vi "cRIO_v5.vi"() -> ()   [LabVIEW 2015]
uses:
  <vilib>/FPGAPlugInAG/cRIO-9113/niLvFpga_Open_cRIO-9113.vi
  <vilib>/rvi/interface/common/dynamic/niFpgaDynamicAddResources.vi
  <vilib>/Utility/error.llb/Error Cluster From Error Code.vi
  <vilib>/FPGAPlugInAG/Dynamic/niLvFpga_Run_Dynamic.vi
  <vilib>/rvi/interface/common/niFpgaWaitOnOcc.vi
  <vilib>/rvi/errors/niLvFpgaAdjustHostInterfaceError.vi
  <vilib>/FPGAPlugInAG/Dynamic/niLvFpga_Close_Dynamic.vi
  <vilib>/rvi/interface/nirviOpenFPGA/nirviOpenFPGA.xnode
  FPGA Bitfiles/DW40ticks_FPGATarget_Fpgav8_YeJ2LnDYWYw.lvbitx
  Fpga_v8.vi
  <vilib>/rvi/interface/nirviMethod/nirviMethod.xnode
  <vilib>/rvi/interface/nirviReadWriteControl/nirviReadWriteControl.xnode
  <vilib>/rvi/interface/nirviCloseFPGA/nirviCloseFPGA.xnode
  <vilib>/rvi/errors/niLvFpgaMergeErrorWithErrorCode.vi
  <vilib>/FPGAPlugInAG/Dynamic/niLvFpga_ReadFifo_Dynamic.vi
  <vilib>/rvi/interface/Simulation/niFpgaSimulationCallBeginRW.vi
  NiFpgaLv.dll
  <vilib>/FPGAPlugInAG/Dynamic/niLvFpga_StartFifo_Dynamic.vi
  <vilib>/FPGAPlugInAG/Dynamic/niLvFpga_ConfigureFifo_Dynamic.vi
panel:
  out "Waveform Graph 4":sgl[](graph)
  out "Waveform Graph 3":sgl[](graph)
  out "Waveform Graph 2":sgl[](graph)
  out "decimated array":i32[](array[numeric])
  out "Analog Input Chart":sgl[][](graph)
  out "Gauge":i16
  out "Aquisition loop rate":u32
  out "error out":errorcluster
  out "Actual Depth of FIFO":u32
  out "Initial write Elements Remaining":u32
  in  "stop":bool
  out "Timed Out?":bool
  out "Number of times timed out":u8
  out "backlog (Elements remaing on the write)":u32
  out "Waveform Graph":sgl[][](graph)
  in  "Data write ON/OFF":bool
  out "Time(ms) for a loop":u32
  in  "start":bool
  out "x-y 3":u32
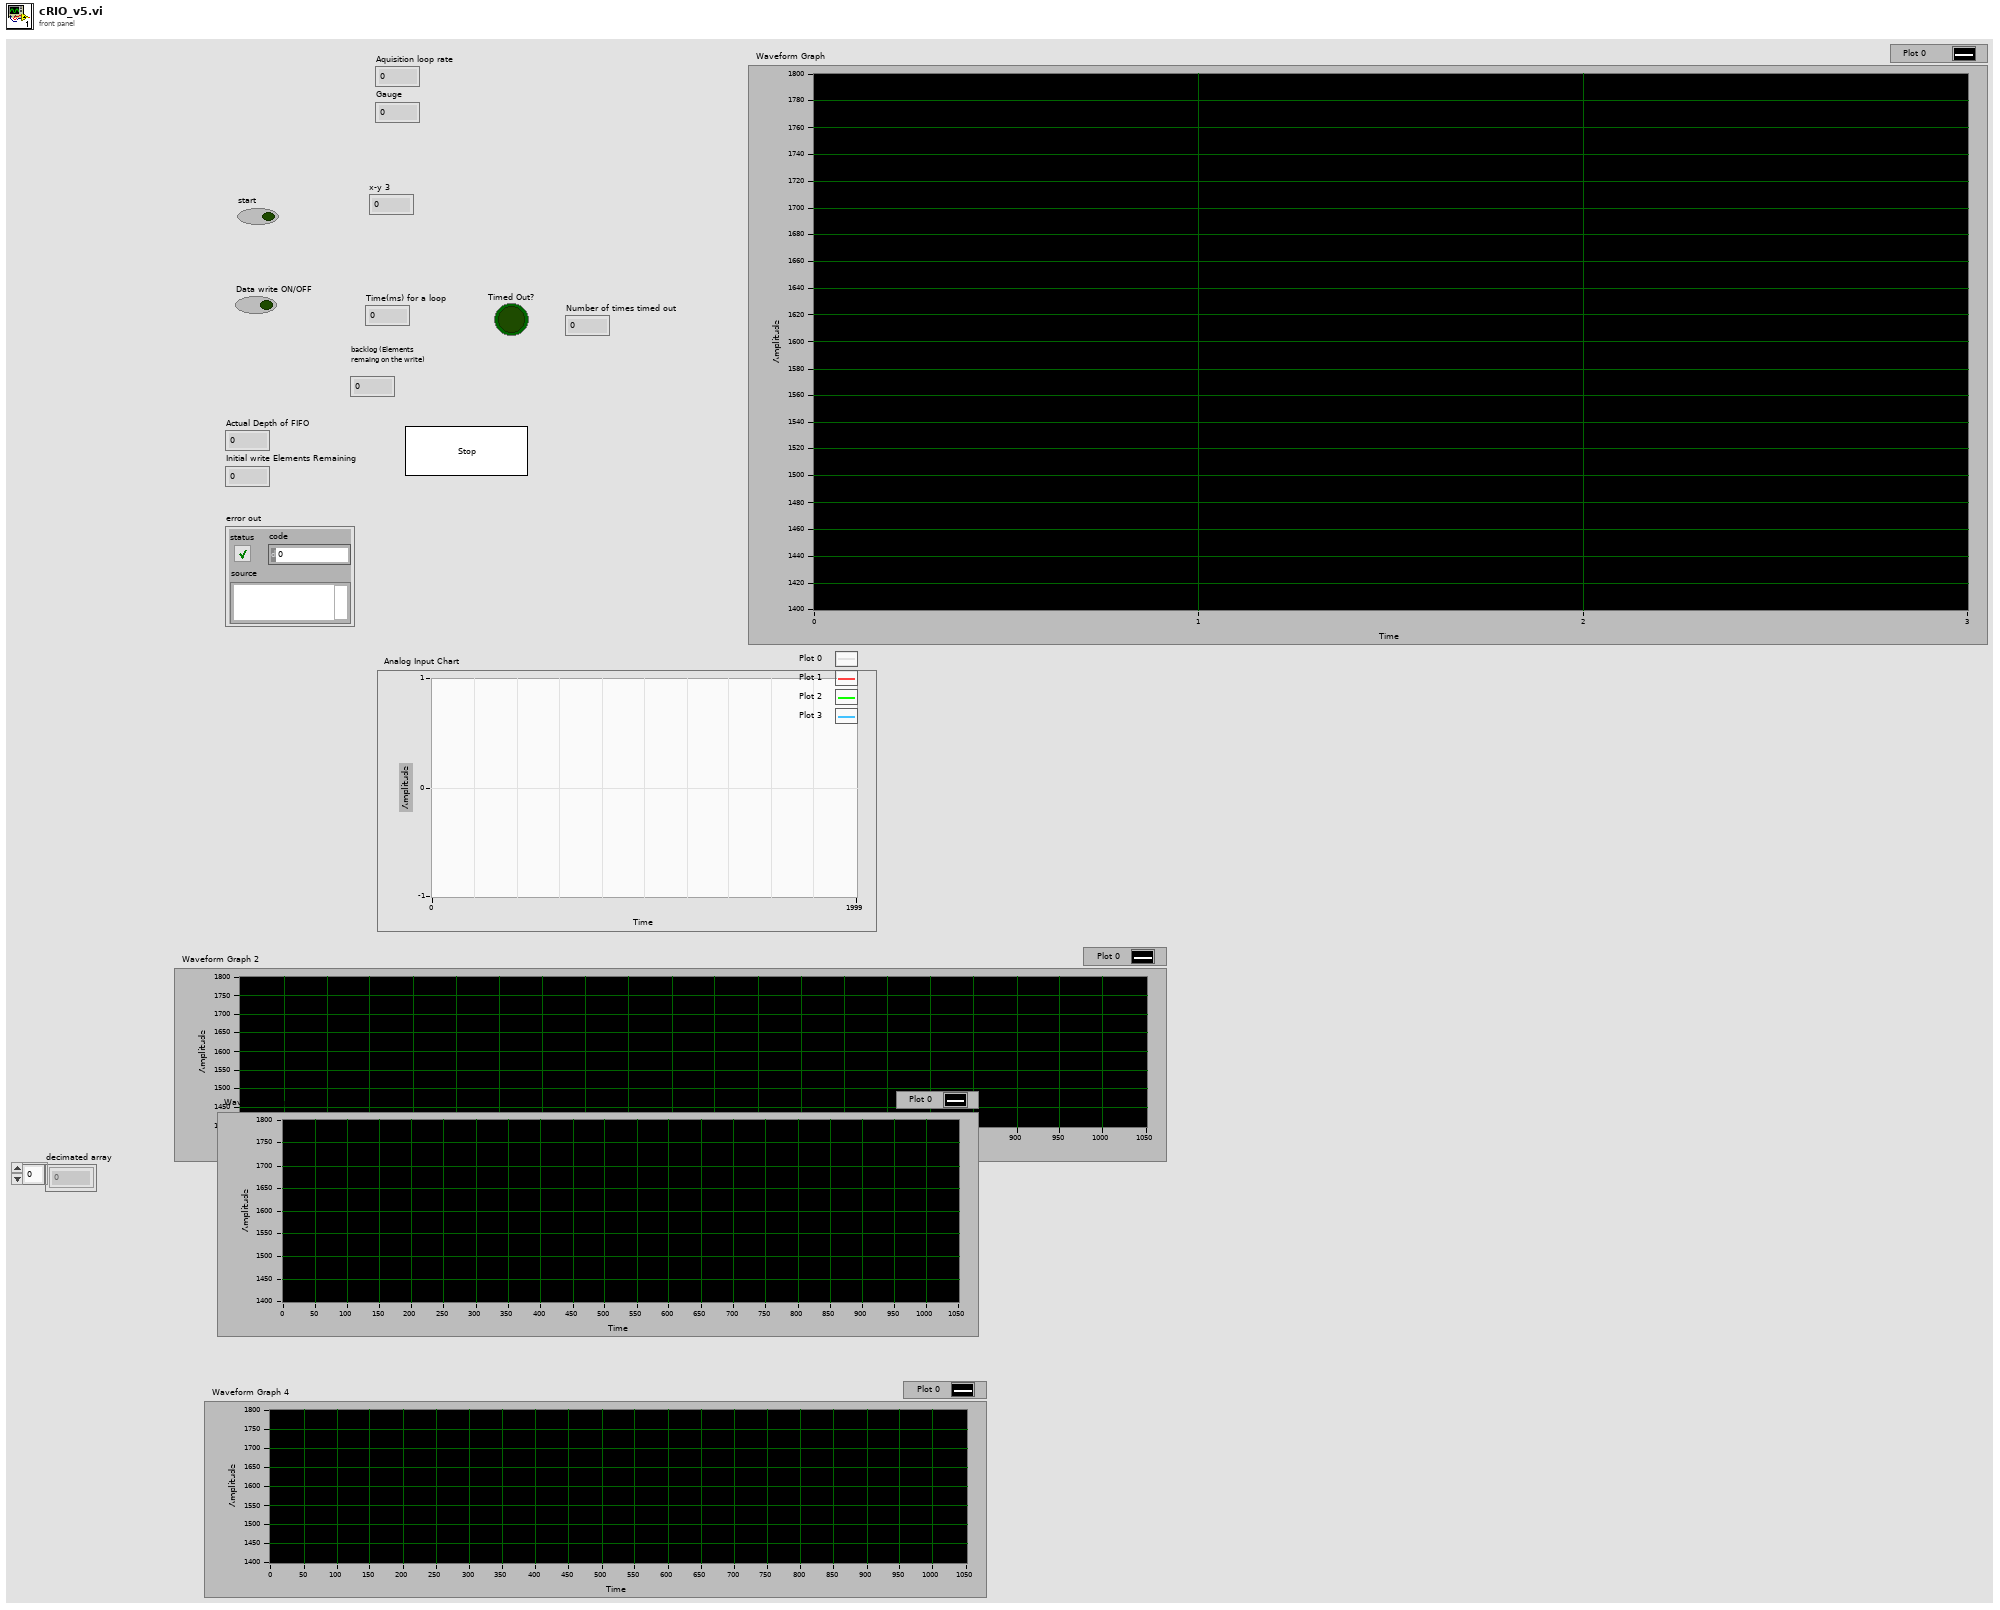
[diagram p1: front panel]
types:
  T1 = enum16{"open", "open or create", "create or replace", "create", "open (read-only)"}
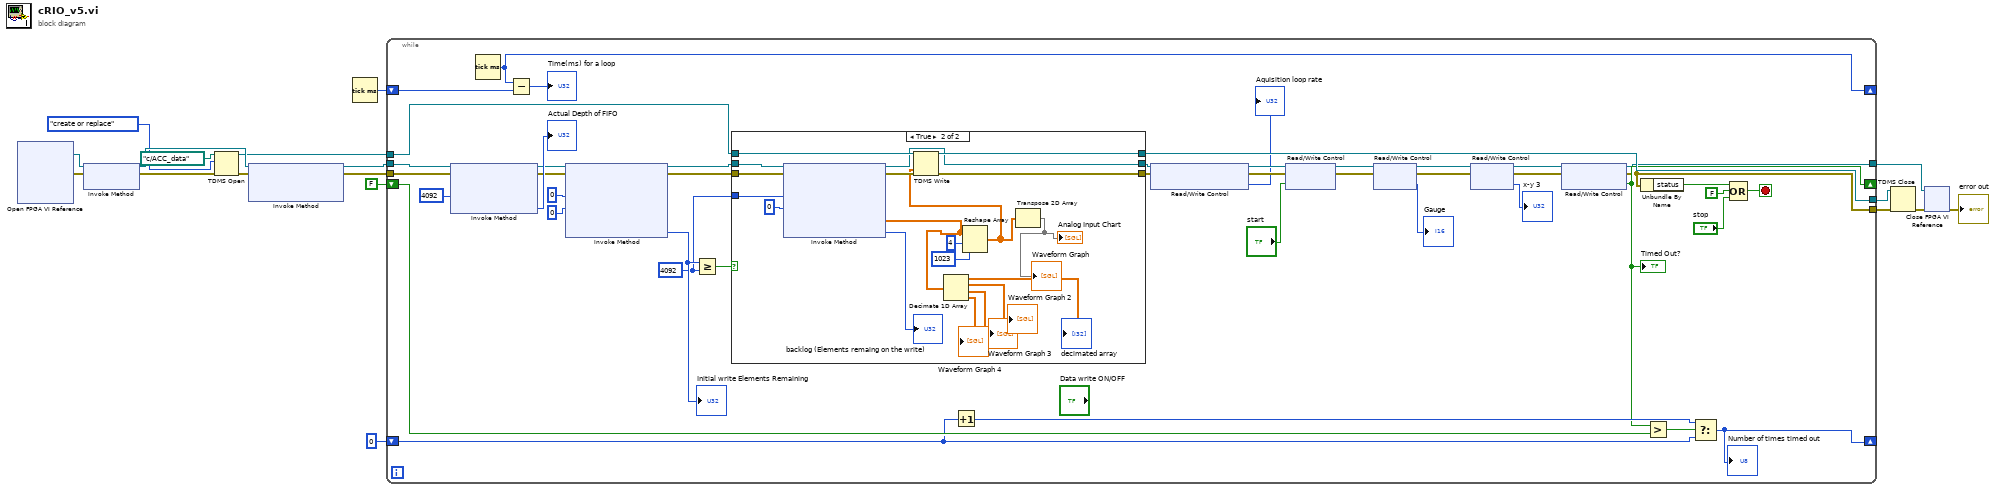
[diagram p0: block diagram]
diagram:
  n1 = xnode "Open FPGA VI Reference"() -> ("FPGA VI Reference Out"=w1:refnum<k20>, "error out"=w2:errorcluster)  [unwired: 2 in]
  n2 = xnode "Invoke Method"("FPGA VI Reference In"=w1, "error in"=w2) -> ("FPGA VI Reference Out"=w17:refnum<k20>, "error out"=w18:errorcluster)
  n3 = TDMS Open(8:w18, 10:T1."create or replace" ("operation (0:open)"), 11:path "c:/ACC_data" ("file path")) -> (0:w16:errorcluster, 3:w11:refnum<k34>)  [unwired: 4 in]
  n4 = xnode "Invoke Method"("FPGA VI Reference In"=w17, "error in"=w16) -> ("FPGA VI Reference Out"=w15:refnum<k20>, "error out"=w14:errorcluster)  [unwired: 1 in]
  n5 = Tick Count (ms)() -> (millisecond timer value=w3:u32)
  n6 = while {
    tunnel: w15 -> [w62]
    tunnel: w14 -> [w61]
    tunnel: w11 -> [w54]
    tunnel: [w52] -> w9
    shift-right: [w38] -> _
    shift-left: FALSE ("Timed Out?") -> [w50]
    shift-right: [w46] -> _
    shift-left: u8 0 -> [w48]
    tunnel: [w33] -> w5
    tunnel: [w32] -> w4
    shift-right: [w36] -> _
    shift-left: w3 -> [w37]
    stop <- w51 stop-if-true
    w41 = u32 4092 ("y")
    n7 = xnode "Invoke Method"("FPGA VI Reference In"=w62, "error in"=w61, "Requested Depth"=u32 4092) -> ("FPGA VI Reference Out"=w59:refnum<k20>, "error out"=w58:errorcluster, "Actual Depth"=→"Actual Depth of FIFO":u32)
    n8 = Tick Count (ms)() -> (millisecond timer value=w36:u32)
    n9 = Subtract(x=w36, y=w37) -> (x-y=→"Time(ms) for a loop":u32)
    n10 = xnode "Invoke Method"("FPGA VI Reference In"=w59, "error in"=w58, "Number of Elements"=u32 0, "Timeout (ms)"=0) -> ("FPGA VI Reference Out"=w42:refnum<k20>, "error out"=w55:errorcluster, "Elements Remaining"=w43:u32)  [unwired: 1 out]
    "Initial write Elements Remaining" <- w43
    n11 = Greater Or Equal?(x=w43, y=w41) -> (x >= y?=w44:bool)
    n12 = case shown="True" w44 {
      tunnel: w55 -> [w63 w80]
      tunnel: w54 -> [w65 w84]
      tunnel: [w63 w83] -> w39
      tunnel: [w65 w82] -> w52
      tunnel: w42 -> [w64 w81]
      tunnel: [w64 w79] -> w40
      tunnel: w41 -> [_ w77]
      frame False {
      }
      frame True {
        n13 = xnode "Invoke Method"("FPGA VI Reference In"=w81, "error in"=w80, "Number of Elements"=w77, "Timeout (ms)"=0) -> ("FPGA VI Reference Out"=w79:refnum<k20>, "error out"=w78:errorcluster, "Data"=w66:sgl[], "Elements Remaining"=→"backlog (Elements remaing on the write)":u32)
        n14 = Decimate 1D Array(w66) -> (→"decimated array":sgl[], →"Waveform Graph 2":sgl[], →"Waveform Graph 3":sgl[], →"Waveform Graph 4":sgl[])
        n15 = Reshape Array(w66, 4 ("dimension size"), 1023 ("dimension size")) -> (w72:sgl[][])
        n16 = TDMS Write(0:w84, 9:w72, 11:w78) -> (4:w82:refnum<k34>, 15:w83:errorcluster)  [unwired: 3 in, 2 out]
        n17 = Transpose 2D Array(2D array=w72) -> (transposed array=→"Waveform Graph" →"Analog Input Chart":sgl[][])
      }
    }
    n18 = Increment(x=w48) -> (x+1=w47:u8)
    n19 = xnode "Read/Write Control"("FPGA VI Reference In"=w40, "error in"=w39) -> ("FPGA VI Reference Out"=w27:refnum<k20>, "error out"=w26:errorcluster, "Aquisition loop rate"=→"Aquisition loop rate":u32)
    n20 = xnode "Read/Write Control"("FPGA VI Reference In"=w27, "error in"=w26, "Boolean"="start") -> ("FPGA VI Reference Out"=w25:refnum<k20>, "error out"=w24:errorcluster)
    n21 = xnode "Read/Write Control"("FPGA VI Reference In"=w25, "error in"=w24) -> ("FPGA VI Reference Out"=w31:refnum<k20>, "error out"=w30:errorcluster, "Gauge"=→"Gauge":i16)
    n22 = xnode "Read/Write Control"("FPGA VI Reference In"=w31, "error in"=w30) -> ("FPGA VI Reference Out"=w28:refnum<k20>, "error out"=w29:errorcluster, "x-y"=→"x-y 3":u32)
    n23 = xnode "Read/Write Control"("FPGA VI Reference In"=w28, "error in"=w29) -> ("FPGA VI Reference Out"=w33:refnum<k20>, "error out"=w32:errorcluster, "Timed Out?"=w38:bool)
    "Timed Out?" <- w38
    n24 = Unbundle By Name(w32) -> ("status"=w45:bool)
    n25 = Greater?(x=w38, y=w50) -> (0:w49:bool)
    n26 = Select(t=w47, s=w49, f=w48) -> (s? t:f=w46:u8)
    "Number of times timed out" <- w46
    n27 = Compound Arithmetic op=OR(w45, FALSE ("value"), "stop") -> (w51:bool)
  }
  n28 = TDMS Close(8:w4, 11:w9) -> (0:w10:errorcluster)  [unwired: 1 out]
  n29 = xnode "Close FPGA VI Reference"("FPGA VI Reference In"=w5, "error in"=w10) -> ("error out"=→"error out":errorcluster)
